vi "all-cubic-spline-test.vi"(8 "error in (no error)":errorcluster) -> (0 "error out":errorcluster, 3 "ALL TESTS PASSED":bool)   [LabVIEW 2019]
panel:
  out "Test 4B":bool
  out "Test 4A":bool
  out "Test 3":bool
  out "Test 2":bool
  out "Test 1":bool
  out "Test 0":bool
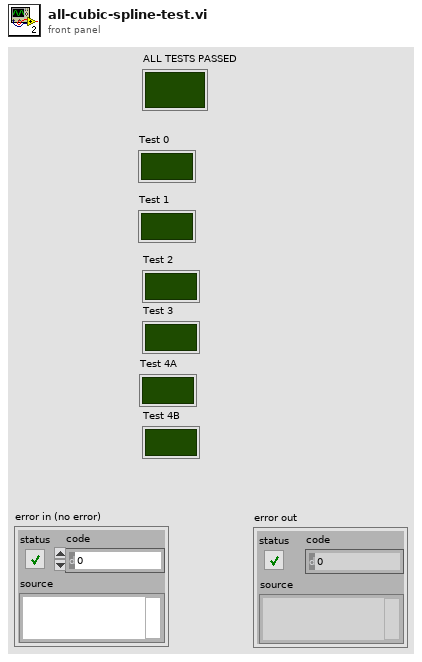
[diagram p1: front panel]
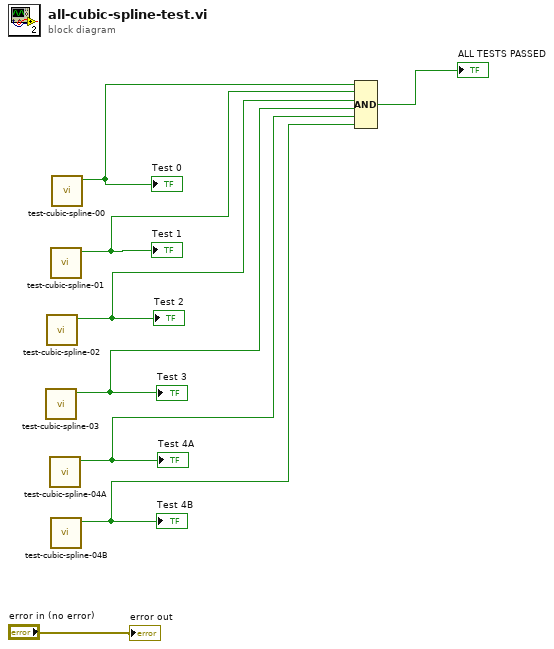
[diagram p0: block diagram]
diagram:
  n1 = call "test-cubic-spline-03.vi"() -> ("Test Passed"=w4:bool)  [unwired: 11 in]
  "Test 3" <- w4
  n2 = call "test-cubic-spline-02.vi"() -> ("Test Passed"=w5:bool)  [unwired: 11 in]
  "Test 2" <- w5
  n3 = call "test-cubic-spline-04A.vi"() -> ("Test Passed"=w3:bool)  [unwired: 11 in]
  "Test 4A" <- w3
  n4 = call "test-cubic-spline-01.vi"() -> ("Test Passed"=w6:bool)  [unwired: 11 in]
  "Test 1" <- w6
  n5 = call "test-cubic-spline-04B.vi"() -> ("Test Passed"=w2:bool)  [unwired: 11 in]
  "Test 4B" <- w2
  n6 = call "test-cubic-spline-00.vi"() -> ("Test Passed"=w7:bool)  [unwired: 11 in]
  "Test 0" <- w7
  n7 = Compound Arithmetic op=AND(w7, w6, w5, w4, w3, w2) -> (→"ALL TESTS PASSED":bool)
  "error out" <- "error in (no error)"
